vi "XL320_Open Motion.vi"(0 "Motor List In":u8[](array[numeric])) -> (4 "Motor List":u8[](array[numeric]), 6 "Motion times":u32[](array[numeric]), 10 "Motion Positions":string[][](table), 14 "File found?":bool, 15 "Speed Scale":dbl)   [LabVIEW 2015]
doc: "Reads a saved Dynamixel Sequence. This VI can also read tab delimitted text files."
uses:
  <instrlib>/Dynamixel XL320/Examples/Record And Playback Motion/Type Defs/XL320_Raw Motion.ctl
  Instance           1 16Saved   OpenFile .vi
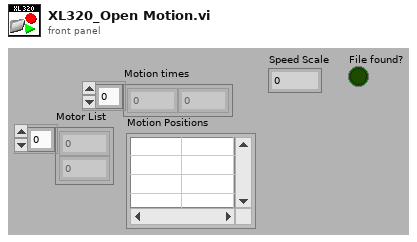
[diagram p1: front panel]
types:
  T1 = typedef "XL320_Raw Motion.ctl" = cluster{"Motor List":u8[], "Gait Positions":string[][], "Gait speeds":u32[], "Speed Scale":dbl}
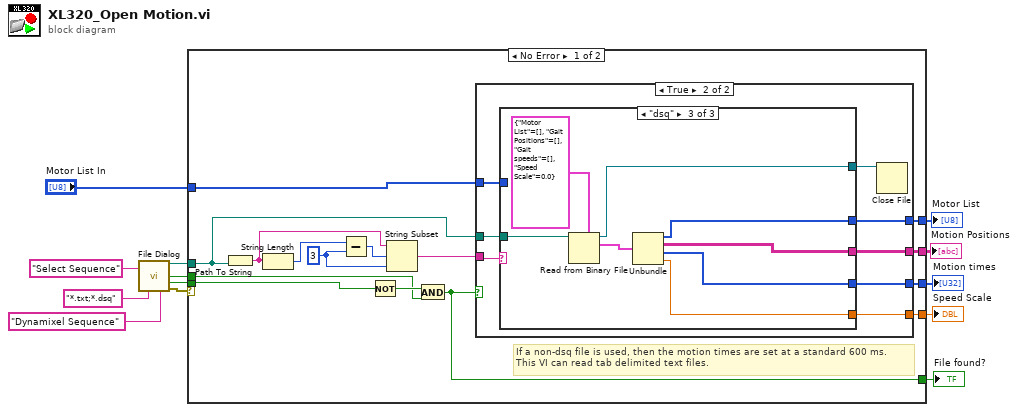
[diagram p0: block diagram]
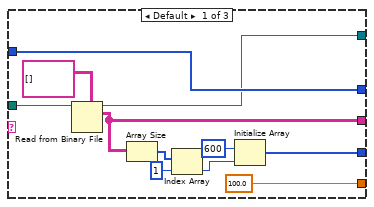
[diagram p3: hidden frame]
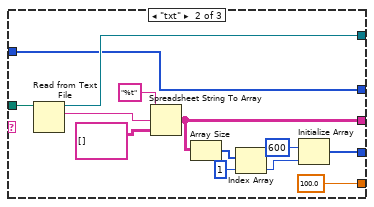
[diagram p4: hidden frame]
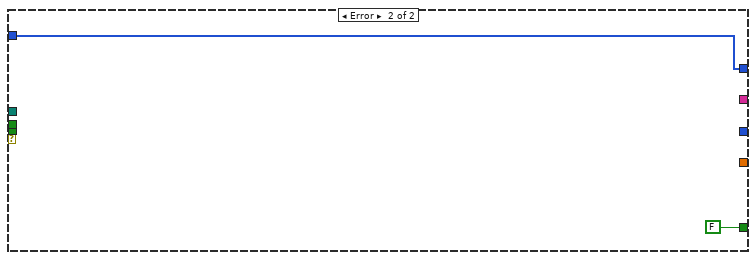
[diagram p5: hidden frame]
diagram:
  n1 = call "File Dialog"("prompt"="Select Sequence", "pattern (all files)"="*.txt;*.dsq", "pattern label"="Dynamixel Sequence") -> ("selected path"=w10:path, "exists"=w8:bool, "cancelled"=w12:bool, "error out"=w1:errorcluster)  [unwired: 9 in]
  n2 = case shown="No Error" w1 {
    tunnel: w12 -> [w28 _]
    tunnel: w10 -> [w27 _]
    tunnel: [w21 _] -> w9
    tunnel: w8 -> [w19 _]
    tunnel: [w18 FALSE] -> w7
    tunnel: [w17 w71] -> w5
    tunnel: [w16 _] -> w4
    tunnel: [w15 _] -> w3
    tunnel: "Motor List In" -> [w14 w71]
    frame No Error {
      w24 = 3 ("length (rest)")
      # "If a non-dsq file is used, then the motion times are set at a standard 600 ms.\nThis VI can read tab delimited text files."
      n3 = Path To String(path=w27) -> (string=w26:string)
      n4 = String Length(string=w26) -> (length=w25:i32)
      n5 = Subtract(x=w25, y=w24) -> (x-y=w23:i32)
      n6 = Not(x=w28) -> (.not. x?=w20:bool)
      n7 = String Subset(string=w26, offset (0)=w23, length (rest)=w24) -> (substring=w22:string)
      n8 = And(x=w20, y=w19) -> (x .and. y?=w18:bool)
      n9 = case shown="True" w18 {
        tunnel: w27 -> [_ w37]
        tunnel: w22 -> [_ w36]
        tunnel: [_ w35] -> w21
        tunnel: [w29 w34] -> w17
        tunnel: [_ w33] -> w16
        tunnel: w14 -> [w29 w31]
        tunnel: [_ w30] -> w15
        frame False {
        }
        frame True {
          n10 = case shown="\"dsq\"" w36 {
            tunnel: w37 -> [w47 w58 w69]
            tunnel: [w41 w53 w66] -> w35
            tunnel: [w48 w50 w67] -> w34
            tunnel: [w40 w52 w65] -> w33
            tunnel: [w38 w51 w64] -> w32
            tunnel: w31 -> [w48 w50 _]
            tunnel: [100.0 ("Speed Scale") 100.0 ("Speed Scale") w63] -> w30
            frame Default {
              n11 = Read from Binary File(5:string[][] [], 11:w47) -> (2:w41:string[][], 3:w38:refnum<file>)  [unwired: 4 in, 2 out]
              n12 = Array Size(array=w41) -> (size(s)=w45:i32[])
              n13 = Index Array(array=w45, index=1) -> (element=w43:i32)
              n14 = Initialize Array(600 ("element"), w43) -> (w40:i32[])
            }
            frame "txt" {
              n15 = Read from Text File(file (use dialog)=w58) -> (refnum out=w51:refnum<file>, text=w61:string)  [unwired: 3 in, 2 out]
              n16 = Spreadsheet String To Array(format string="%t", spreadsheet string=w61, array type (2D Dbl)=string[][] []) -> (array=w53:string[][])  [unwired: 1 in]
              n17 = Array Size(array=w53) -> (size(s)=w57:i32[])
              n18 = Index Array(array=w57, index=1) -> (element=w55:i32)
              n19 = Initialize Array(u32 600 ("element"), w55) -> (w52:u32[])
            }
            frame "dsq" {
              n20 = Read from Binary File(5:T1 {"Motor List"=[], "Gait Positions"=[], "Gait speeds"=[], "Speed Scale"=0.0} ("Raw Motion"), 11:w69) -> (2:w68:T1, 3:w64:refnum<file>)  [unwired: 4 in, 2 out]
              n21 = Unbundle(w68) -> ("Motor List"=w67:u8[], "Gait Positions"=w66:string[][], "Gait speeds"=w65:u32[], "Speed Scale"=w63:dbl)
            }
          }
          n22 = Close File(refnum=w32) -> ()  [unwired: 1 in, 2 out]
        }
      }
    }
    frame Error {
    }
  }
  "Motion Positions" <- w9
  "File found?" <- w7
  "Motion times" <- w4
  "Motor List" <- w5
  "Speed Scale" <- w3
